vi "Encode Password.vi"(8 "error in (no error)":errorcluster, 10 "Plain Password":string, 11 "BasicPasswordEncoder in":refnum<class "BasicPasswordEncoder.lvclass">) -> (0 "error out":errorcluster, 2 "Encoded Password":string, 3 "BasicPasswordEncoder out":refnum<class "BasicPasswordEncoder.lvclass">)   [LabVIEW 2020, in "HTTP Server.lvlib" / "BasicPasswordEncoder.lvclass"]
uses:
  BasicPasswordEncoder.lvclass
  lv-web-crypto/lv-crypto/Crypto/Crypto.lvlib
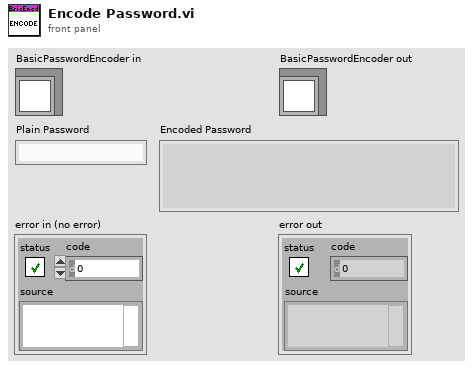
[diagram p1: front panel]
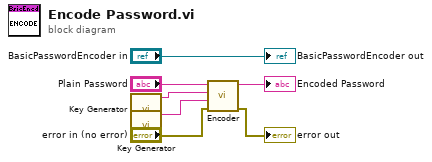
[diagram p0: block diagram]
diagram:
  n1 = call "Key Generator.vi"() -> ("Key"=w5:string)  [unwired: 10 in, 1 out]
  n2 = call "Key Generator.vi"() -> ("Key"=w4:string)  [unwired: 10 in, 1 out]
  n3 = call "Encoder.vi"("error in (no error)"="error in (no error)", "Salt 2"=w4, "Salt 1"=w5, "Plain Password"="Plain Password") -> ("error out"=→"error out":errorcluster, "Encoded Password"=→"Encoded Password":string)  [unwired: 6 in]
  "BasicPasswordEncoder out" <- "BasicPasswordEncoder in"
